vi "PulseDetect80AndSwitch160_60.vi"(6 "Switch for":i32=6, 8 "Fill from last":i32=6, 9 "Laser bits in":bool[](array[boolean])=[FALSE, FALSE, FALSE, FALSE, FALSE, FALSE, FALSE, FALSE, FALSE, FALSE, FALSE, FALSE, FALSE, FALSE, FALSE, FALSE, FALSE, FALSE, FALSE, FALSE, FALSE, FALSE, FALSE, FALSE, FALSE, FALSE, FALSE, FALSE, FALSE, FALSE, FALSE, FALSE, FALSE, FALSE, FALSE, FALSE, FALSE, FALSE, FALSE, FALSE, FALSE, FALSE, FALSE, FALSE, FALSE, FALSE, FALSE, FALSE, FALSE, FALSE, FALSE, FALSE, FALSE, FALSE, FALSE, FALSE, FALSE, FALSE, FALSE, FALSE], 10 "Last area in":bool, 11 "Last laser bit in":bool) -> (0 "Fill after last":i32=6, 1 "Area bits out":bool[](array[boolean]), 2 "New last area out":bool, 3 "New last laser bit out":bool)   [LabVIEW 2012]
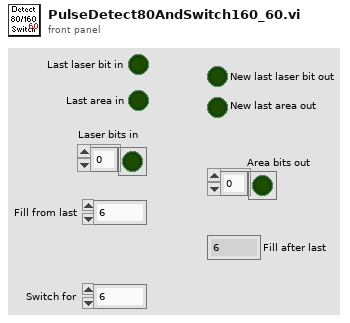
[diagram p1: front panel]
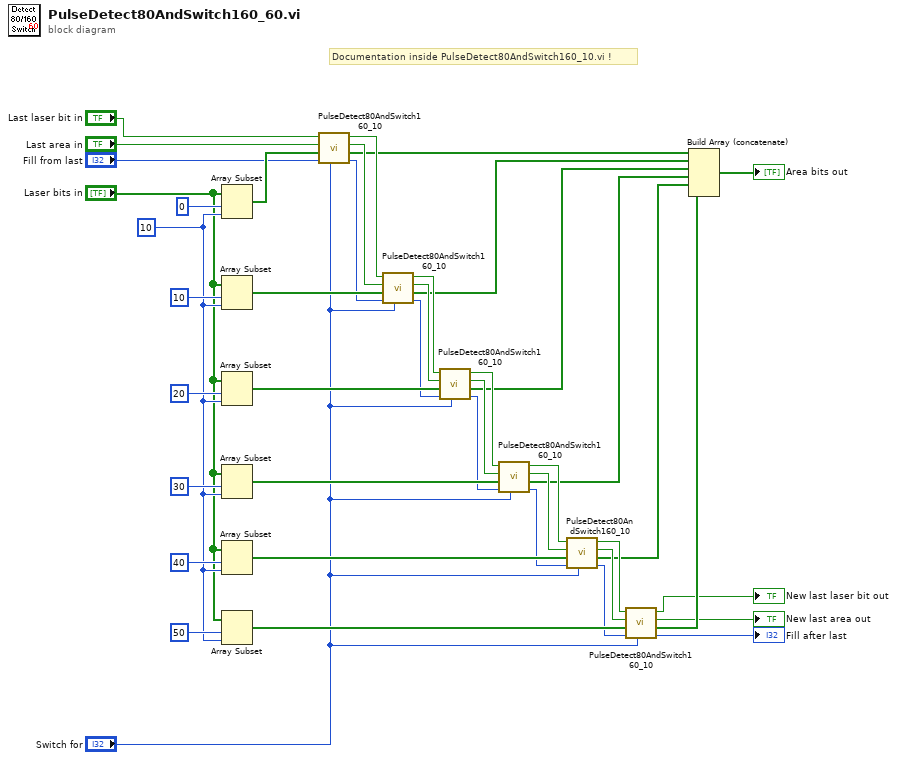
[diagram p0: block diagram]
diagram:
  w34 = 10 ("length")
  # "Documentation inside PulseDetect80AndSwitch160_10.vi !"
  n1 = Array Subset(array="Laser bits in", index=0, length=w34) -> (w40:bool[])
  n2 = Array Subset(array="Laser bits in", index=10, length=w34) -> (w30:bool[])
  n3 = Array Subset(array="Laser bits in", index=20, length=w34) -> (w27:bool[])
  n4 = Array Subset(array="Laser bits in", index=30, length=w34) -> (w23:bool[])
  n5 = Array Subset(array="Laser bits in", index=40, length=w34) -> (w17:bool[])
  n6 = Array Subset(array="Laser bits in", index=50, length=w34) -> (w15:bool[])
  n7 = call "PulseDetect80AndSwitch160_10.vi"("Switch for"="Switch for", "Fill from last"="Fill from last", "Laser bits in"=w40, "Last area in"="Last area in", "Last laser bit in"="Last laser bit in") -> ("Fill after last"=w28:i32, "Area array out"=w11:bool[], "New last area out"=w31:bool, "New last laser bit out"=w32:bool)  [unwired: 3 in]
  n8 = call "PulseDetect80AndSwitch160_10.vi"("Switch for"="Switch for", "Fill from last"=w28, "Laser bits in"=w30, "Last area in"=w31, "Last laser bit in"=w32) -> ("Fill after last"=w24:i32, "Area array out"=w10:bool[], "New last area out"=w25:bool, "New last laser bit out"=w26:bool)  [unwired: 3 in]
  n9 = call "PulseDetect80AndSwitch160_10.vi"("Switch for"="Switch for", "Fill from last"=w24, "Laser bits in"=w27, "Last area in"=w25, "Last laser bit in"=w26) -> ("Fill after last"=w20:i32, "Area array out"=w9:bool[], "New last area out"=w21:bool, "New last laser bit out"=w22:bool)  [unwired: 3 in]
  n10 = call "PulseDetect80AndSwitch160_10.vi"("Switch for"="Switch for", "Fill from last"=w20, "Laser bits in"=w23, "Last area in"=w21, "Last laser bit in"=w22) -> ("Fill after last"=w16:i32, "Area array out"=w8:bool[], "New last area out"=w18:bool, "New last laser bit out"=w19:bool)  [unwired: 3 in]
  n11 = call "PulseDetect80AndSwitch160_10.vi"("Switch for"="Switch for", "Fill from last"=w16, "Laser bits in"=w17, "Last area in"=w18, "Last laser bit in"=w19) -> ("Fill after last"=w12:i32, "Area array out"=w7:bool[], "New last area out"=w13:bool, "New last laser bit out"=w14:bool)  [unwired: 3 in]
  n12 = call "PulseDetect80AndSwitch160_10.vi"("Switch for"="Switch for", "Fill from last"=w12, "Laser bits in"=w15, "Last area in"=w13, "Last laser bit in"=w14) -> ("Fill after last"=→"Fill after last":i32, "Area array out"=w6:bool[], "New last area out"=→"New last area out":bool, "New last laser bit out"=→"New last laser bit out":bool)  [unwired: 3 in]
  n13 = Build Array (concatenate)(w11, w10, w9, w8, w7, w6) -> (→"Area bits out":bool[])
